vi "Write test data to file_old.vi"(0 "imei":string="ImeiImeiImeiIme", 1 "Meid":string="MediMeidMeidMe", 3 "Pass date time":string="12-06-2014 10:05:00", 4 "SIM ID":string="SimSimSimSimSimSimID", 5 "Mac":string="MacMacMacMac", 7 "phone":string="ImeiImeiImeiIme", 9 "Serial Number":string="SerialNum", 11 "error in (no error)":errorcluster, 14 "Style":string="100060") -> (10 "PassFail":string="Fail", 15 "error out":errorcluster)   [LabVIEW 2013]
uses:
  Main Support/Global 2.vi
  Test Globals/Global 1.vi
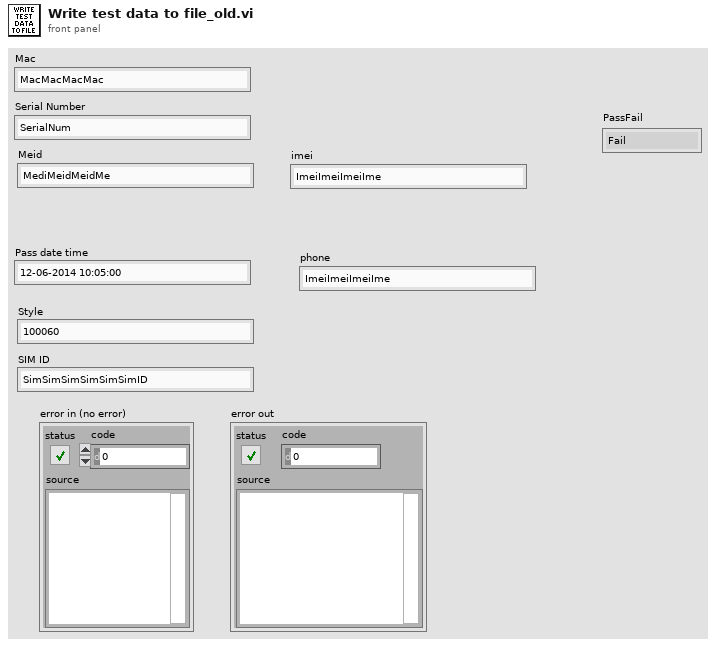
[diagram p1: front panel]
types:
  T1 = enum16{"open", "replace", "create", "open or create", "replace or create", "replace or create with confirmation"}
  T2 = enum16{"get next serial number available", "change status to assigned", "change status to available", "change status to tentative"}
  T3 = cluster{"Test folder":string, "Top level":string, "Main":string, "Test report":string, "Work order qty":string, "Work order meid":string, "Work order imei":string, "Master meid imei list":string, "Master test data":string, "ZPL label info":string, "Pictures":string, "Setup info":string, "Work order":string, "Tests folder":string, "Tests steps folder":string, "Config folder":string, "Verizon Upload file":string, "Job data file":string, "Station globals":string, "Post test info":string}
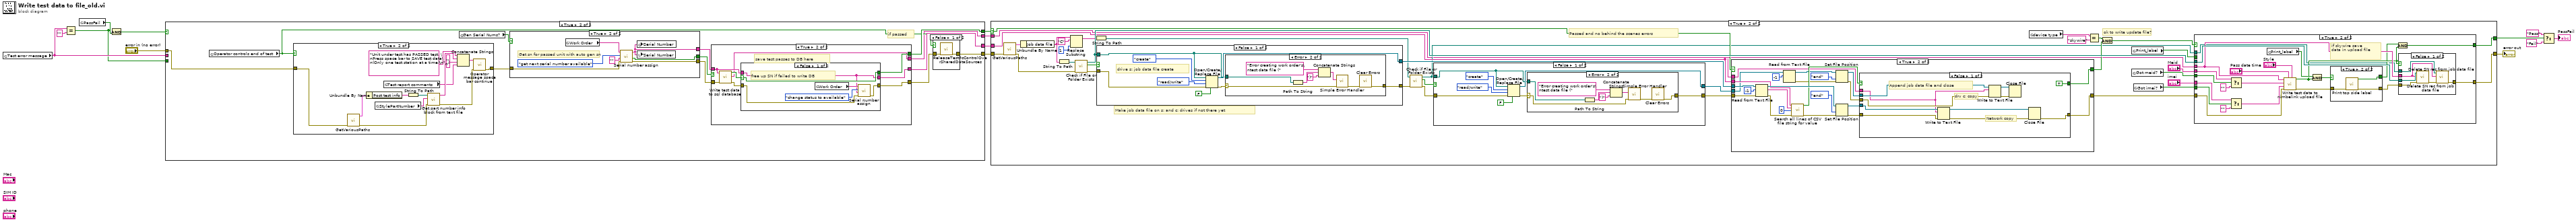
[diagram p0: block diagram]
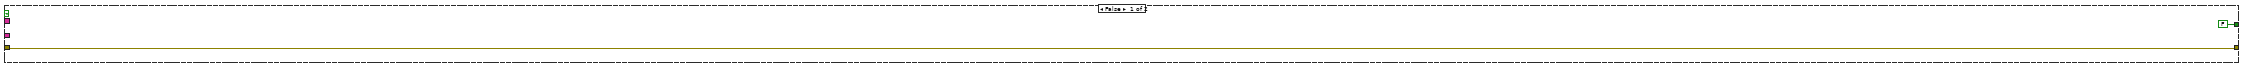
[diagram p2: hidden frame]
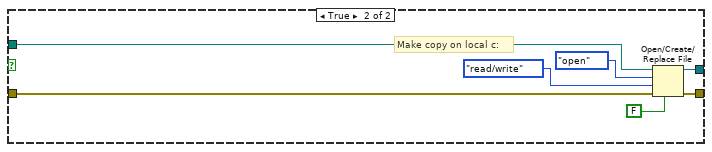
[diagram p4: hidden frame]
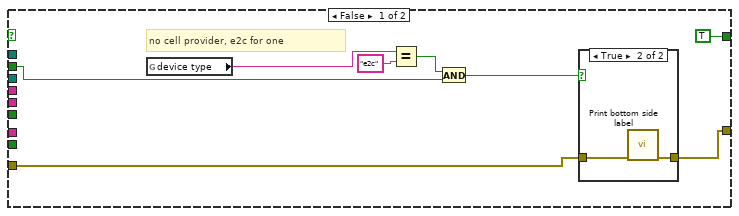
[diagram p5: hidden frame]
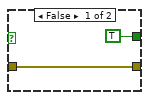
[diagram p7: hidden frame]
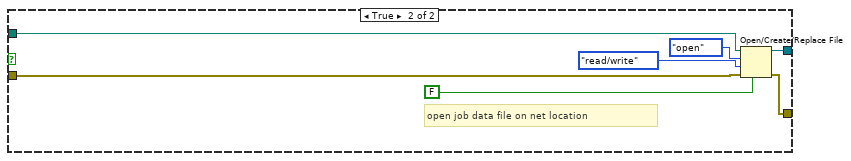
[diagram p10: hidden frame]
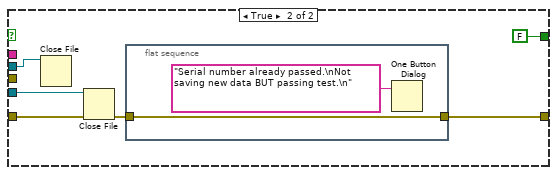
[diagram p12: hidden frame]
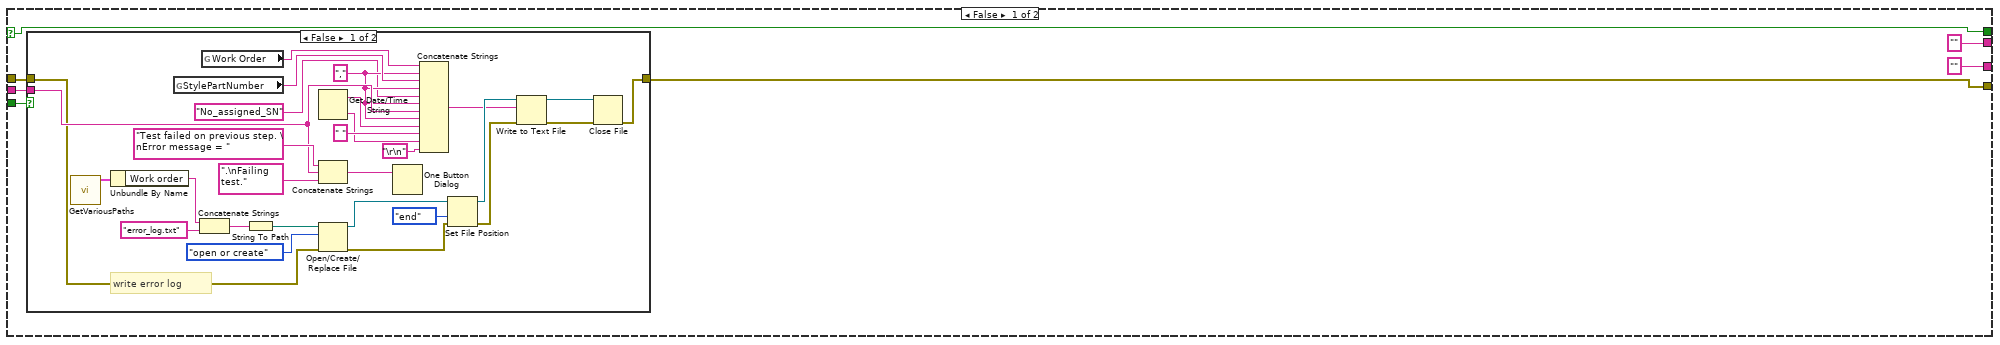
[diagram p13: hidden frame]
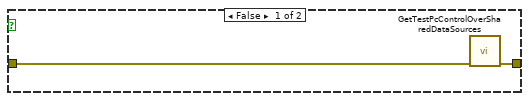
[diagram p16: hidden frame]
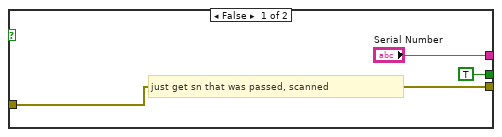
[diagram p17: hidden frame]
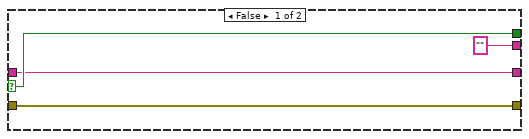
[diagram p18: hidden frame]
diagram:
  n1 = global read "Global 1.vi" "Test error message"() -> (w4:string)
  n2 = Equal?(x=w4, y="") -> (x = y?=w3:bool)
  n3 = global read "Global 2.vi" "PassFail"() -> (w6:bool)
  n4 = And(x=w3, y=w6) -> (x .and. y?=w5:bool)
  n5 = case shown="True" w5 {
    selector: w5 -> [w22 _]
    tunnel: [w16 w54] -> w8
    tunnel: "error in (no error)" -> [w17 w57]
    tunnel: [w22 w63] -> w9
    tunnel: w4 -> [w21 _]
    tunnel: w3 -> [w20 _]
    tunnel: ["" ("Serial number out") w58] -> w2
    tunnel: ["" ("Test rec csv line") w52] -> w1
    frame False {
      n6 = case shown="False" w20 {
        tunnel: w21 -> [w37 _]
        tunnel: w17 -> [w26 w51]
        tunnel: [w25 w51] -> w16
        frame False {
          w36 = "," ("string")
          # "write error log"
          n7 = call "GetVariousPaths.vi"() -> ("Built Paths"=w47:T3)  [unwired: 10 in, 1 out]
          n8 = Unbundle By Name(w47) -> ("Work order"=w46:string)
          n9 = global read "Global 2.vi" "StylePartNumber"() -> (w38:string)
          n10 = Concatenate Strings(w46, "error_log.txt" ("string")) -> (w24:string)
          n11 = global read "Global 2.vi" "Work Order"() -> (w39:string)
          n12 = String To Path(string=w24) -> (path=w44:path)
          n13 = Get Date/Time String() -> (date string=w35:string, time string=w33:string)  [unwired: 3 in]
          n14 = Concatenate Strings("Test failed on previous step. \nError message = " ("string"), w37, ".\nFailing test." ("string")) -> (w50:string)
          n15 = Open/Create/Replace File(file path (use dialog)=w44, error in=w26, operation (0:open)=T1."open or create") -> (refnum out=w41:refnum<file>, error out=w42:errorcluster)  [unwired: 3 in, 1 out]
          n16 = One Button Dialog(message=w50) -> ()  [unwired: 1 in, 1 out]
          n17 = Concatenate Strings(w39, w36, w38, w36, "No_assigned_SN" ("string"), w36, w37, w36, w35, " " ("string"), w33, "\r\n") -> (w29:string)
          n18 = Set File Position(refnum=w41, from (0:start)=enum16{"start", "end", "current"}."end", error in=w42) -> (refnum out=w31:refnum<file>, error out=w30:errorcluster)  [unwired: 1 in]
          n19 = Write to Text File(file (use dialog)=w31, text=w29, error in=w30) -> (refnum out=w27:refnum<file>, error out=w28:errorcluster)  [unwired: 1 in, 1 out]
          n20 = Close File(refnum=w27, error in=w28) -> (error out=w25:errorcluster)  [unwired: 1 out]
        }
        frame True {
        }
      }
    }
    frame True {
      # "if passed"
      n21 = global read "Global 2.vi" "Operator controls end of test"() -> (w53:bool)
      n22 = case shown="True" w53 {
        tunnel: w57 -> [w68 w72]
        tunnel: [w67 w71] -> w56
        frame False {
          n23 = call "GetTestPcControlOverSharedDataSources.vi"("error in (no error)"=w68) -> ("error out"=w67:errorcluster)  [unwired: 10 in]
        }
        frame True {
          n24 = call "GetVariousPaths.vi"("error in (no error)"=w72) -> ("error out"=w75:errorcluster, "Built Paths"=w81:T3)  [unwired: 9 in]
          n25 = Unbundle By Name(w81) -> ("Post test info"=w78:string)
          n26 = global read "Global 2.vi" "StylePartNumber"() -> (w76:string)
          n27 = global read "Global 1.vi" "Test report comments"() -> (w69:string)
          n28 = String To Path(string=w78) -> (path=w77:path)
          n29 = call "Get part number info block from text file.vi"("error in (no error)"=w75, "StylePartNum"=w76, "file (use dialog)"=w77) -> ("error out"=w74:errorcluster, "Info block"=w73:string)  [unwired: 6 in, 1 out]
          n30 = Concatenate Strings("Unit under test has PASSED test. \nPress space bar to SAVE test data\n(Only one test station at a time)\n" ("Message"), w73, "\n" ("string"), w69) -> (w79:string)
          n31 = call "Operator message space bar continue.vi"("error in (no error)"=w74, "Message"=w79) -> ("error out"=w71:errorcluster)  [unwired: 9 in]
        }
      }
      n32 = global read "Global 1.vi" "Gen Serial Nums?"() -> (w60:bool)
      n33 = case shown="True" w60 {
        tunnel: w56 -> [w83 w86]
        tunnel: [w83 w90] -> w62
        tunnel: ["Serial Number" w87] -> w59
        tunnel: [TRUE ("Got serial number?") w85] -> w61
        frame False {
          # "just get sn that was passed, scanned"
        }
        frame True {
          # "Get sn for passed unit with auto gen sn"
          n34 = global read "Global 2.vi" "Work Order"() -> (w88:string)
          n35 = call "Serial number assign.vi"("Error in (no error)"=w86, "Serial number in"="", "Operation"=T2."get next serial number available", "Work order"=w88) -> ("Error out"=w90:errorcluster, "OK?"=w85:bool, "Serial number out"=w87:string)  [unwired: 5 in]
          n36 = global write "Global 2.vi" "Serial Number"(w87) -> ()
          n37 = local write "Serial Number"(w87) -> ()
        }
      }
      n38 = case shown="True" w61 {
        selector: w61 -> [w95 _]
        tunnel: [w94 w100] -> w55
        tunnel: [w95 w98] -> w63
        tunnel: w62 -> [w94 w103]
        tunnel: w59 -> [w93 w99]
        tunnel: [w93 w97] -> w58
        tunnel: ["" ("Test rec csv line") w96] -> w52
        frame False {
        }
        frame True {
          # "save test passes to DB here"
          n39 = call "Write test data to sql database.vi"("error in (no error)"=w103, "Serial"=w99) -> ("error out"=w101:errorcluster, "Test rec csv line"=w96:string, "Passed?"=w102:bool)  [unwired: 5 in]
          n40 = case shown="False" w102 {
            selector: w102 -> [w105 w111]
            tunnel: w101 -> [w109 w112]
            tunnel: [w108 w112] -> w100
            tunnel: w99 -> [w104 w110]
            tunnel: [w105 w111] -> w98
            tunnel: [w104 w110] -> w97
            frame False {
              # "free up SN if failed to write DB"
              n41 = global read "Global 2.vi" "Work Order"() -> (w107:string)
              n42 = call "Serial number assign.vi"("Error in (no error)"=w109, "Serial number in"=w104, "Operation"=T2."change status to available", "Work order"=w107) -> ("Error out"=w108:errorcluster)  [unwired: 5 in, 2 out]
            }
            frame True {
            }
          }
        }
      }
      n43 = case shown="False" w53 {
        tunnel: w55 -> [w65 w66]
        tunnel: [w64 w66] -> w54
        frame False {
          n44 = call "ReleaseTestPcControlOverSharedDataSources.vi"("error in (no error)"=w65) -> ("error out"=w64:errorcluster)  [unwired: 10 in]
        }
        frame True {
        }
      }
    }
  }
  n45 = case shown="True" w9 {
    selector: w9 -> [_ w138]
    tunnel: [FALSE ("Write OK?") w147] -> w12
    tunnel: w8 -> [w114 w142]
    tunnel: [w114 w141] -> w10
    tunnel: w2 -> [_ w137]
    tunnel: w1 -> [_ w117]
    frame False {
    }
    frame True {
      # "Make job data file on s: and c: drives if not there yet"
      # "ok to write update file?"
      # "Passed and no behind the scenes errors"
      n46 = call "GetVariousPaths.vi"("error in (no error)"=w142) -> ("error out"=w129:errorcluster, "Built Paths"=w149:T3)  [unwired: 9 in]
      n47 = Unbundle By Name(w149) -> ("Job data file"=w116:string)
      n48 = String To Path(string=w116) -> (path=w127:path)
      n49 = Replace Substring(2:1 ("length (len. of substring)"), 4:"C" ("substring (\"\")"), 5:w116) -> (1:w115:string)  [unwired: 1 in, 1 out]
      n50 = call <vilib>:"Check if File or Folder Exists.vi"("error in (no error)"=w129, "path"=w127) -> ("error out"=w145:errorcluster, "file or folder exists?"=w146:bool, "dup path"=w143:path)  [unwired: 7 in]
      n51 = String To Path(string=w115) -> (path=w124:path)
      n52 = case shown="False" w146 {
        tunnel: w143 -> [w219 w242]
        tunnel: w145 -> [w225 w240]
        tunnel: [w220 w239] -> w120
        tunnel: [w223 w241] -> w144
        frame False {
          # "drive s: job data file create"
          n53 = Open/Create/Replace File(file path (use dialog)=w219, error in=w225, operation (0:open)=T1."create", access (0:read/write)=enum16{"read/write", "read-only", "write-only"}."read/write", disable buffering (F)=FALSE) -> (refnum out=w223:refnum<file>, error out=w221:errorcluster)  [unwired: 1 in, 1 out]
          n54 = case shown="Error" w221 {
            selector: w221 -> [w227 w230]
            tunnel: [w227 w235] -> w220
            tunnel: w219 -> [_ w232]
            frame No Error {
            }
            frame Error {
              n55 = Path To String(path=w232) -> (string=w231:string)
              n56 = Concatenate Strings("Error creating work order's\ntest data file (" ("message"), w231, ")" ("string")) -> (w228:string)
              n57 = call <vilib>:"Simple Error Handler.vi"("error source (\" \")"=w228, "error in (no error)"=w230) -> ("error out"=w229:errorcluster)  [unwired: 3 in, 4 out]
              n58 = call <vilib>:"Clear Errors.vi"("error in (no error)"=w229) -> ("error out"=w235:errorcluster)  [unwired: 6 in]
            }
          }
        }
        frame True {
          # "open job data file on net location"
          n59 = Open/Create/Replace File(file path (use dialog)=w242, error in=w240, operation (0:open)=T1."open", access (0:read/write)=enum16{"read/write", "read-only", "write-only"}."read/write", disable buffering (F)=FALSE) -> (refnum out=w241:refnum<file>, error out=w239:errorcluster)  [unwired: 1 in, 1 out]
        }
      }
      n60 = call <vilib>:"Check if File or Folder Exists.vi"("error in (no error)"=w120, "path"=w124) -> ("error out"=w119:errorcluster, "file or folder exists?"=w123:bool, "dup path"=w121:path)  [unwired: 7 in]
      n61 = case shown="False" w123 {
        tunnel: w121 -> [w150 w173]
        tunnel: w119 -> [w156 w171]
        tunnel: [w151 w170] -> w118
        tunnel: [w154 w172] -> w122
        frame False {
          n62 = Open/Create/Replace File(file path (use dialog)=w150, error in=w156, operation (0:open)=T1."create", access (0:read/write)=enum16{"read/write", "read-only", "write-only"}."read/write", disable buffering (F)=FALSE) -> (refnum out=w154:refnum<file>, error out=w152:errorcluster)  [unwired: 1 in, 1 out]
          n63 = case shown="Error" w152 {
            selector: w152 -> [w158 w163]
            tunnel: [w158 w166] -> w151
            tunnel: w150 -> [_ w161]
            frame No Error {
            }
            frame Error {
              n64 = Path To String(path=w161) -> (string=w160:string)
              n65 = Concatenate Strings("Error creating work order's\ntest data file (" ("message"), w160, ")" ("string")) -> (w159:string)
              n66 = call <vilib>:"Simple Error Handler.vi"("error source (\" \")"=w159, "error in (no error)"=w163) -> ("error out"=w162:errorcluster)  [unwired: 3 in, 4 out]
              n67 = call <vilib>:"Clear Errors.vi"("error in (no error)"=w162) -> ("error out"=w166:errorcluster)  [unwired: 6 in]
            }
          }
        }
        frame True {
          # "Make copy on local c:"
          n68 = Open/Create/Replace File(file path (use dialog)=w173, error in=w171, operation (0:open)=T1."open", access (0:read/write)=enum16{"read/write", "read-only", "write-only"}."read/write", disable buffering (F)=FALSE) -> (refnum out=w172:refnum<file>, error out=w170:errorcluster)  [unwired: 1 in, 1 out]
        }
      }
      n69 = case shown="True" w138 {
        selector: w138 -> [w243 _]
        tunnel: w144 -> [_ w261]
        tunnel: w137 -> [_ w257]
        tunnel: w118 -> [w244 w262]
        tunnel: [w244 w254] -> w148
        tunnel: [w243 w253] -> w139
        tunnel: w122 -> [_ w249]
        tunnel: w117 -> [_ w245]
        frame False {
        }
        frame True {
          n70 = Read from Text File(file (use dialog)=w261, count=-1, error in=w262) -> (refnum out=w265:refnum<file>, text=w258:string, error out=w260:errorcluster)  [unwired: 1 in, 1 out]
          n71 = Read from Text File(file (use dialog)=w249, count=-1) -> (refnum out=w252:refnum<file>, error out=w247:errorcluster)  [unwired: 2 in, 2 out]
          n72 = call "Search all lines of CSV file string for value.vi"("Compare value"=w257, "CSV file string"=w258, "CSV field (0-n)"=0, "error in"=w260) -> ("Found value"=w255:bool, "error out"=w259:errorcluster)  [unwired: 10 in]
          n73 = Set File Position(refnum=w252, from (0:start)=enum16{"start", "end", "current"}."end", error in=w247) -> (refnum out=w248:refnum<file>, error out=w246:errorcluster)  [unwired: 1 in]
          n74 = Set File Position(refnum=w265, from (0:start)=enum16{"start", "end", "current"}."end", error in=w259) -> (refnum out=w264:refnum<file>, error out=w263:errorcluster)  [unwired: 1 in]
          n75 = case shown="False" w255 {
            tunnel: w264 -> [w277 w283]
            tunnel: w263 -> [w278 w284]
            tunnel: [w276 w281] -> w254
            tunnel: [TRUE FALSE] -> w253
            tunnel: w248 -> [w270 w279]
            tunnel: w246 -> [w269 _]
            tunnel: w245 -> [w268 _]
            frame False {
              # "Network copy"
              # "drv c: copy"
              # "Append job data file and close"
              n76 = Write to Text File(file (use dialog)=w277, text=w268, error in=w278) -> (refnum out=w274:refnum<file>, error out=w275:errorcluster)  [unwired: 1 in, 1 out]
              n77 = Write to Text File(file (use dialog)=w270, text=w268, error in=w269) -> (refnum out=w272:refnum<file>, error out=w271:errorcluster)  [unwired: 1 in, 1 out]
              n78 = Close File(refnum=w272, error in=w271) -> ()  [unwired: 2 out]
              n79 = Close File(refnum=w274, error in=w275) -> (error out=w276:errorcluster)  [unwired: 1 out]
            }
            frame True {
              n80 = Close File(refnum=w279) -> ()  [unwired: 1 in, 2 out]
              n81 = Close File(refnum=w283, error in=w284) -> (error out=w282:errorcluster)  [unwired: 1 out]
              n82 = flat-sequence {
                tunnel: w282 -> [w286]
                tunnel: [w286] -> w281
                frame #0 {
                  n83 = One Button Dialog(message="Serial number already passed.\nNot saving new data BUT passing test.\n") -> ()  [unwired: 1 in, 1 out]
                }
              }
            }
          }
        }
      }
      n84 = global read "Global 1.vi" "device type"() -> (w131:string)
      n85 = Equal?(x=w131, y="skywire") -> (x = y?=w130:bool)
      n86 = And(x=w130, y=w139) -> (x .and. y?=w140:bool)
      n87 = global read "Global 1.vi" "Print_label"() -> (w133:bool)
      n88 = global read "Global 1.vi" "Got meid?"() -> (w128:bool)
      n89 = global read "Global 1.vi" "Got imei?"() -> (w134:bool)
      n90 = case shown="True" w140 {
        tunnel: w148 -> [w176 w206]
        tunnel: [w175 w205] -> w141
        tunnel: w137 -> [_ w203]
        tunnel: [TRUE ("Write OK?") w187] -> w147
        tunnel: w143 -> [_ w204]
        tunnel: "Meid" -> [_ w195]
        tunnel: "imei" -> [_ w192]
        tunnel: w134 -> [_ w191]
        tunnel: w133 -> [w174 _]
        tunnel: w128 -> [_ w186]
        tunnel: w121 -> [_ w185]
        frame False {
          # "no cell provider, e2c for one"
          n91 = global read "Global 1.vi" "device type"() -> (w180:string)
          n92 = Equal?(x=w180, y="e2c") -> (x = y?=w178:bool)
          n93 = And(x=w178, y=w174) -> (x .and. y?=w177:bool)
          n94 = case shown="True" w177 {
            tunnel: w176 -> [w182 w184]
            tunnel: [w182 w183] -> w175
            frame False {
            }
            frame True {
              n95 = call "Print bottom side label.vi"("error in (no error)"=w184) -> ("error out"=w183:errorcluster)  [unwired: 7 in, 1 out]
            }
          }
        }
        frame True {
          # "if skywire save\ndata in upload file"
          n96 = Select(t=w195, s=w186, f="") -> (s? t:f=w194:string)
          n97 = Select(t=w192, s=w191, f="") -> (s? t:f=w190:string)
          n98 = global read "Global 1.vi" "Print_label"() -> (w202:bool)
          n99 = call "Write test data to nimbelink upload file.vi"("Style"="Style", "Pass date time"="Pass date time", "error in (no error)"=w206, "imei"=w190, "Meid"=w194, "Serial Number"=w203) -> ("error out"=w200:errorcluster, "Write OK?"=w189:bool)  [unwired: 1 in, 1 out]
          n100 = And(x=w202, y=w189) -> (x .and. y?=w201:bool)
          n101 = case shown="True" w201 {
            tunnel: w200 -> [w208 w211]
            tunnel: [w208 w210] -> w199
            tunnel: [TRUE ("Print Label OK?") w209] -> w188
            frame False {
            }
            frame True {
              n102 = call "Print top side label.vi"("error in (no error)"=w211) -> ("error out"=w210:errorcluster, "Print Label OK?"=w209:bool)  [unwired: 7 in]
            }
          }
          n103 = And(x=w188, y=w189) -> (x .and. y?=w187:bool)
          n104 = case shown="False" w189 {
            tunnel: w199 -> [w217 w218]
            tunnel: [w212 w218] -> w205
            tunnel: w204 -> [w216 _]
            tunnel: w203 -> [w215 _]
            tunnel: w185 -> [w214 _]
            frame False {
              n105 = call "Delete SN rec from job data file.vi"("error in"=w217, "Serial number"=w215, "file (use dialog)"=w216) -> ("error out"=w213:errorcluster)  [unwired: 8 in]
              n106 = call "Delete SN rec from job data file.vi"("error in"=w213, "Serial number"=w215, "file (use dialog)"=w214) -> ("error out"=w212:errorcluster)  [unwired: 8 in]
            }
            frame True {
            }
          }
        }
      }
    }
  }
  "error out" <- w10
  n107 = Select(t="Pass", s=w12, f="Fail") -> (s? t:f=→"PassFail":string)
